vi "Bidirectional Streaming RouteGuide Test.vi"() -> ()   [LabVIEW 2019, in "route_guide_client.lvlib"]
uses:
  route_guide_client.lvlib
  RPC Messages/routeguide_RouteNote.ctl
  RPC Messages/routeguide_Point.ctl
  <vilib>/gRPC/LabVIEW gRPC Library/grpc-lvsupport-release.lvlib
panel:
  out "error out":errorcluster
  out "Response Data":T1[](array[typedef])
  in  "Request Data":T1[](array[typedef])=[{"location"={"latitude"=1, "longitude"=1}, "message"="Point 1"}, {"location"={"latitude"=2, "longitude"=2}, "message"="Point 2"}]
  in  "Server Address":string="localhost:50051"
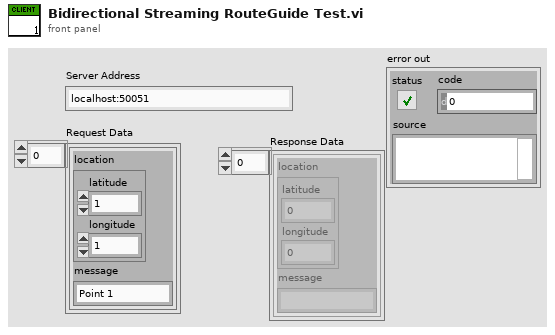
[diagram p1: front panel]
types:
  T1 = typedef "route_guide_client.lvlib/routeguide_RouteNote.ctl" = cluster{"location":T2, "message":string}
  T2 = typedef "route_guide_client.lvlib/routeguide_Point.ctl" = cluster{"latitude":i32, "longitude":i32}
  T3 = typedef "grpc-lvsupport-release.lvlib/grpcId.ctl" = u64
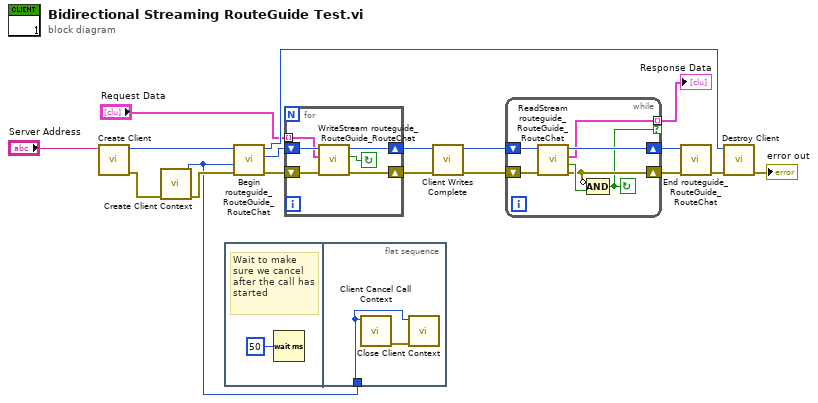
[diagram p0: block diagram]
diagram:
  n1 = call "Create Client.vi"("address"="Server Address") -> ("error out"=w4:errorcluster, "gRPC ID Out"=w17:T3)  [unwired: 9 in]
  n2 = call <vilib>:"Create Client Context.vi"("error in (no error)"=w4) -> ("error out"=w3:errorcluster, "ContextID out"=w2:T3)  [unwired: 9 in]
  n3 = flat-sequence {
    tunnel: w2 -> [w20]
    frame #0 {
      # "Wait to make sure we cancel after the call has started"
      n4 = Wait (ms)(milliseconds to wait=u32 50) -> ()  [unwired: 1 out]
    }
    frame #1 {
      n5 = call <vilib>:"Client Cancel Call Context.vi"("Call ID in"=w20) -> ("error out"=w21:errorcluster)  [unwired: 10 in]
      n6 = call <vilib>:"Close Client Context.vi"("error in (no error)"=w21, "ContextID"=w20) -> ()  [unwired: 9 in, 1 out]
    }
  }
  n7 = call "Begin routeguide_RouteGuide_RouteChat.vi"("error in"=w3, "contextId"=w2, "gRPC ID"=w17) -> ("error out"=w15:errorcluster, "Call Id Out"=w16:T3, "gRPC ID out"=w13:T3)  [unwired: 6 in]
  n8 = for {
    shift-right: [w24] -> w8
    shift-left: w16 -> [w27]
    shift-right: [w23] -> w6
    shift-left: w15 -> [w26]
    tunnel: "Request Data" -> [w25] mode=indexing
    stop <- w22 continue-if-true
    n9 = call "WriteStream routeguide_RouteGuide_RouteChat.vi"("error in"=w26, "Request Data"=w25, "Call ID in"=w27) -> ("error out"=w23:errorcluster, "Success"=w22:bool, "Call ID"=w24:T3)  [unwired: 6 in]
  }
  n10 = call <vilib>:"Client Writes Complete.vi"("error in"=w6, "ClientID in"=w8) -> ("error out"=w5:errorcluster, "ClientID out"=w7:T3)  [unwired: 8 in]
  n11 = while {
    shift-right: [w30] -> w11
    shift-left: w7 -> [w33]
    shift-right: [w31] -> w10
    shift-left: w5 -> [w32]
    tunnel: [w29] -> w9 mode=indexing if=w28
    stop <- w28 continue-if-true
    n12 = call "ReadStream routeguide_RouteGuide_RouteChat.vi"("error in"=w32, "Call ID in"=w33) -> ("error out"=w31:errorcluster, "Success"=w34:bool, "Response Data"=w29:T1, "Call ID"=w30:T3)  [unwired: 6 in]
    n13 = Compound Arithmetic op=AND(invert w31, w34) -> (w28:bool)
  }
  "Response Data" <- w9
  n14 = call "End routeguide_RouteGuide_RouteChat.vi"("error in"=w10, "Call ID in"=w11) -> ("error out"=w14:errorcluster)  [unwired: 8 in, 1 out]
  n15 = call "Destroy Client.vi"("error in"=w14, "gRPC ID"=w13) -> ("error out"=→"error out":errorcluster)  [unwired: 9 in]
